vi "main.vi"() -> ()   [LabVIEW 2018]
uses:
  <vilib>/vision/Pattern Matching.llb/IMAQ Curve Parameters.ctl
  Classes/EdgeDetectionProcessor/private/Curvature Data STYP.ctl
  Classes/EdgeDetectionProcessor/EdgeDetectionProcessor.lvclass
  C:/Program Files/National Instruments/LabVIEW 2018/user.lib/Aaron/File IO/Video/Video Processor/Video Processor.lvclass
  <vilib>/vision/NI_Vision_Development_Module.lvlib
panel:
  in  "Curvature Threshold":dbl
  out "Curvatures":T1[](array[typedef])
  in  "stop":bool
  in  "Curve Parameters":T2={"Extraction Mode"=0, "Edge Threshold"=75, "Edge Filter Size"=1, "Min Length"=25, "Row Search Step Size"=15, "Col Search Step Size"=15, "Max Endpoint Gap"=10, "Closed"=FALSE, "Subpixel"=FALSE} {"Max Endpoint Gap" min=0; "Col Search Step Size" min=1 max=255 step=1; "Row Search Step Size" min=1 max=255 step=1; "Min Length" min=0; "Edge Filter Size" items=["Fine", "Normal", "Controur Tracing"]; "Edge Threshold" min=1 max=65535 step=1; "Extraction Mode" items=["Normal", "Uniform Regions"]}
  out "Frame":i32
  out "Image":T3(plugin-control)
  in  "Path":path
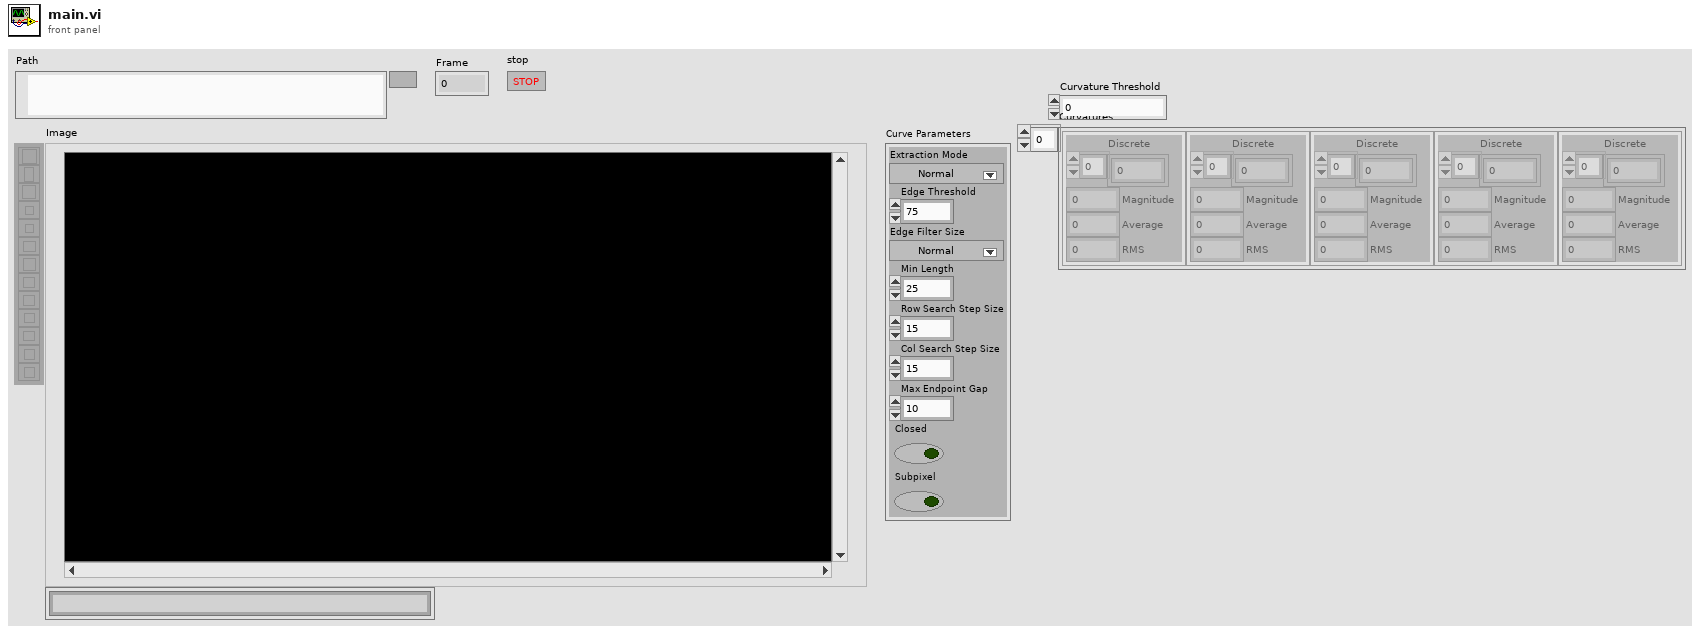
[diagram p1: front panel]
types:
  T1 = typedef "EdgeDetectionProcessor.lvclass/Curvature Data STYP.ctl" = cluster{"Discrete":dbl[], "Magnitude":dbl, "Average":dbl, "RMS":dbl}
  T2 = typedef "IMAQ Curve Parameters.ctl" = cluster{"Extraction Mode":u32, "Edge Threshold":i32, "Edge Filter Size":u32, "Min Length":i32, "Row Search Step Size":i32, "Col Search Step Size":i32, "Max Endpoint Gap":i32, "Closed":bool, "Subpixel":bool}
  T3 = typedef "IMAQ Image.ctl" = refnum<image>
  T4 = typedef "Image Type" = u32
  T5 = typedef "IMAQ ExtractCurvesCurve.ctl" = cluster{"Points":cluster{"X":dbl, "Y":dbl}[], "Closed?":bool, "Curve Length":dbl, "Min Edge Strength":dbl, "Max Edge Strength":dbl, "Average Edge Strength":dbl}
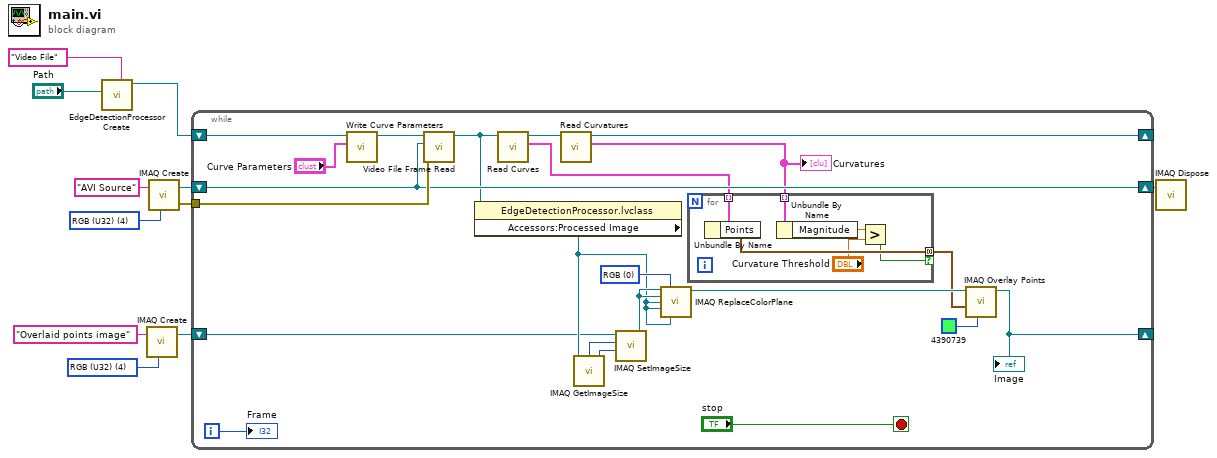
[diagram p0: block diagram]
diagram:
  w2 = T4 4 items=["Grayscale (U8)", "Grayscale (I16)", "Grayscale (SGL)", "Complex (CSG)", "RGB (U32)", "HSL (U32)", "RGB (U64)", "Grayscale (U16)"] ("Image Type")
  w7 = T4 4 items=["Grayscale (U8)", "Grayscale (I16)", "Grayscale (SGL)", "Complex (CSG)", "RGB (U32)", "HSL (U32)", "RGB (U64)", "Grayscale (U16)"] ("Image Type")
  n1 = call "EdgeDetectionProcessor Create.vi"("Identifier"="Video File", "Path"="Path") -> ("EdgeDetectionProcessor out"=w9:refnum<class "EdgeDetectionProcessor.lvclass">)  [unwired: 8 in, 1 out]
  n2 = call "IMAQ Create"("Image Name"="Overlaid points image", "Image Type"=w2) -> ("New Image"=w1:T3)  [unwired: 3 in, 1 out]
  n3 = call "IMAQ Create"("Image Name"="AVI Source", "Image Type"=w7) -> ("New Image"=w6:T3, "error out"=w5:errorcluster)  [unwired: 3 in]
  n4 = while {
    shift-right: [w13] -> _
    shift-left: w9 -> [w29]
    tunnel: w5 -> [w32]
    shift-right: [w31] -> w4
    shift-left: w6 -> [w31]
    shift-right: [w15] -> _
    shift-left: w1 -> [w16]
    i -> [w33]
    stop <- "stop" stop-if-true
    w25 = u16 0 items=["RGB", "HSL", "HSV", "HSI"] ("Color Mode")
    n5 = call-dynamic "Write Curve Parameters.vi"("Curve Parameters"="Curve Parameters", "EdgeDetectionProcessor in"=w29) -> ("EdgeDetectionProcessor out"=w28:refnum<class "EdgeDetectionProcessor.lvclass">)  [unwired: 8 in, 1 out]
    n6 = call-dynamic "Video File Frame Read.vi"("error in (no error)"=w32, "Image Dst"=w31, "Video Processor in"=w28) -> ("Video Processor out"=w27:refnum<class "EdgeDetectionProcessor.lvclass">)  [unwired: 4 in, 4 out]
    n7 = property class="EdgeDetectionProcessor.lvclass"(reference=w27) -> ("Accessors:Processed Image"=w19:T3)  [unwired: 1 in, 2 out]
    n8 = call-dynamic "Read Curves.vi"("EdgeDetectionProcessor in"=w27) -> ("Curves"=w22:T5[], "EdgeDetectionProcessor out"=w14:refnum<class "EdgeDetectionProcessor.lvclass">)  [unwired: 8 in, 1 out]
    n9 = call-dynamic "Read Curvatures.vi"("EdgeDetectionProcessor in"=w14) -> ("Curvatures"=w12:T1[], "EdgeDetectionProcessor out"=w13:refnum<class "EdgeDetectionProcessor.lvclass">)  [unwired: 8 in, 1 out]
    "Curvatures" <- w12
    n10 = call "IMAQ GetImageSize"("Image"=w19) -> ("Y Resolution"=w17:i32, "X Resolution"=w18:i32)  [unwired: 3 in, 1 out]
    n11 = call "IMAQ SetImageSize"("Y Resolution"=w17, "X Resolution"=w18, "Image"=w16) -> ("Image Out"=w20:T3)  [unwired: 2 in, 1 out]
    n12 = call "IMAQ ReplaceColorPlane"("Image Src"=w20, "Color Mode"=w25, "Image Dst"=w20, "Red or Hue Plane"=w19, "Green or Sat Plane"=w19, "Blue or Luma or Val or Inten Plane"=w19) -> ("Image Dst Out"=w24:T3)  [unwired: 8 in, 1 out]
    n13 = for {
      tunnel: w22 -> [w39] mode=indexing
      tunnel: [w38] -> w21 mode=concatenating if=w35
      tunnel: w12 -> [w37] mode=indexing
      n14 = Unbundle By Name(w39) -> ("Points"=w38:cluster{"X":dbl, "Y":dbl}[])
      n15 = Unbundle By Name(w37) -> ("Magnitude"=w36:dbl)
      n16 = Greater?(x=w36, y="Curvature Threshold") -> (0:w35:bool)
    }
    n17 = call "IMAQ Overlay Points"("Color"=u32 4390739, "Array of Points"=w21, "Image"=w24) -> ("Image Out"=w15:T3)  [unwired: 7 in, 1 out]
    "Image" <- w15
    "Frame" <- w33
  }
  n18 = call "IMAQ Dispose"("Image"=w4) -> ()  [unwired: 5 in, 1 out]
